vi "serial_read.vi"(0 "FPGA I/O In":refnum<k21>="RMC/DIO2", 1 "FIFO In":refnum<k21>="Serial read 1", 2 "tick/2 every bit":u32, 3 "tick every bit":u32) -> ()   [LabVIEW 2012]
uses:
  <vilib>/rvi/eio/common/nirviEmuTemplateMethod_errors.vi
  <vilib>/rvi/DataTransferAndStorage/Container/Common/niFpgaContainerExecOnDevCompGetState.vi
  <vilib>/rvi/Emulation/niFpgaSctlEmulationGetInTimedLoop.vi
  <vilib>/rvi/DataTransferAndStorage/Container/Common/niFpgaContainerGetUniqueNameForEmu.vi
  <vilib>/rvi/FIFO/Fifo_Resource/nirvififoEmulationSetSize.vi
  <vilib>/rvi/errors/niFpgaSetErrorForExecOnDevCompSimple.vi
  <vilib>/rvi/eio/common/nirviEmuReportErrorAndStop.vi
  <vilib>/rvi/Emulation/niFpgaSctlEmulationFifoFullMgr.vi
  <vilib>/rvi/Emulation/niFpgaSctlEmulationResourceMgr.vi
  <vilib>/rvi/interface/RandomDataEmulation/nirviRandomDataFPGAFIFO.vi
  <vilib>/rvi/interface/RandomDataEmulation/niFpgaRandomDataHandleErrors.vi
  <vilib>/eio/EIONode/EIONode.xnode
  <vilib>/rvi/DataTransferAndStorage/Container/XNode/niFpgaContainer.xnode
  <vilib>/rvi/FIFO/Fifo_Resource/niFpgaFifoEmulationRefIn.vi
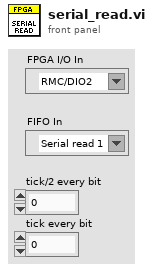
[diagram p1: front panel]
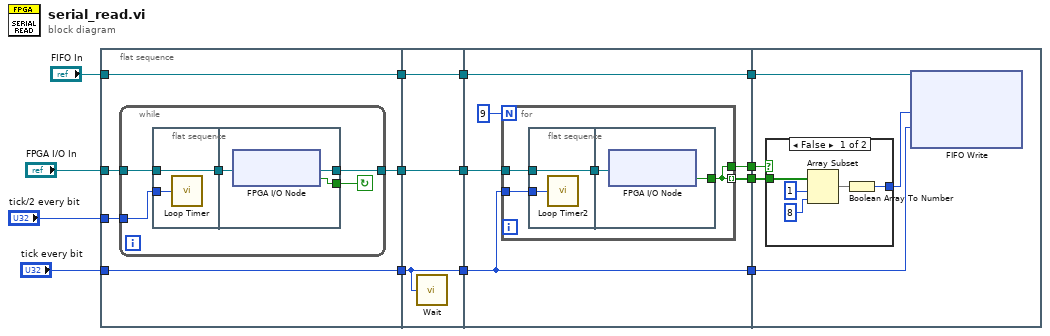
[diagram p0: block diagram]
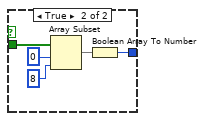
[diagram p2: hidden frame]
diagram:
  n1 = flat-sequence {
    tunnel: "FIFO In" -> [w17]
    tunnel: "FPGA I/O In" -> [w19]
    tunnel: [w18] -> w10
    tunnel: [w17] -> w9
    tunnel: "tick/2 every bit" -> [w16]
    tunnel: [w15] -> w8
    tunnel: "tick every bit" -> [w15]
    tunnel: w10 -> [w32]
    tunnel: [w32] -> w7
    tunnel: w9 -> [w31]
    tunnel: [w31] -> w6
    tunnel: w8 -> [w30]
    tunnel: [w30] -> w5
    tunnel: w7 -> [w37]
    tunnel: [w36] -> w4
    tunnel: [w35] -> w3
    tunnel: w6 -> [w34]
    tunnel: [w34] -> w2
    tunnel: w5 -> [w33]
    tunnel: [w33] -> w1
    tunnel: w4 -> [w51]
    tunnel: w3 -> [w50]
    tunnel: w2 -> [w49]
    tunnel: w1 -> [w47]
    frame #0 {
      n2 = while {
        tunnel: w19 -> [w24]
        tunnel: [w22] -> w18
        tunnel: w16 -> [w20]
        stop <- w23 continue-if-true
        n3 = flat-sequence {
          tunnel: w24 -> [w26]
          tunnel: [w26] -> w21
          tunnel: w20 -> [w25]
          tunnel: [w28] -> w23
          tunnel: [w27] -> w22
          tunnel: w21 -> [w29]
          frame #0 {
            n4 = call "Loop Timer"("Count(Ticks)"=w25) -> ()  [unwired: 1 out]
          }
          frame #1 {
            n5 = xnode "FPGA I/O Node"("FPGA I/O In"=w29) -> ("I/O Item"=w28:bool, "FPGA I/O Out"=w27:refnum<k21>)
          }
        }
      }
    }
    frame #1 {
      n6 = call "Wait"("Count(Ticks)"=w30) -> ()  [unwired: 1 out]
    }
    frame #2 {
      n7 = for {
        N: 9 -> [_]
        tunnel: w37 -> [w42]
        tunnel: [w40] -> w35 mode=indexing
        tunnel: [w40] -> w36
        tunnel: w33 -> [w39]
        n8 = flat-sequence {
          tunnel: w42 -> [w44]
          tunnel: [w44] -> w41
          tunnel: w39 -> [w43]
          tunnel: [w45] -> w40
          tunnel: w41 -> [w46]
          frame #0 {
            n9 = call "Loop Timer2"("Count(Ticks)"=w43) -> ()  [unwired: 1 out]
          }
          frame #1 {
            n10 = xnode "FPGA I/O Node"("FPGA I/O In"=w46) -> ("I/O Item"=w45:bool)  [unwired: 1 out]
          }
        }
      }
    }
    frame #3 {
      n11 = case shown="False" w51 {
        tunnel: w50 -> [w53 w61]
        tunnel: [w52 w57] -> w48
        frame False {
          n12 = Array Subset(array=w53, index=1, length=8) -> (w54:bool[])
          n13 = Boolean Array To Number(Boolean array=w54) -> (number=w52:u8)
        }
        frame True {
          n14 = Array Subset(array=w61, index=0, length=8) -> (w58:bool[])
          n15 = Boolean Array To Number(Boolean array=w58) -> (number=w57:u8)
        }
      }
      n16 = xnode ("FIFO Write")("Element"=w48, "Timeout"=w47, "FIFO In"=w49) -> ()  [unwired: 2 out]
    }
  }
